vi "SetSMOState.vi"(8 "error in (no error)":errorcluster, 10 "SMO State":T1, 11 "SMO in":refnum<class "SMO.lvclass">) -> (0 "error out":errorcluster, 3 "SMO out":refnum<class "SMO.lvclass">)   [LabVIEW 2021, in "smo.lvlib" / "SMO.lvclass"]
uses:
  SMO.lvclass
  Typedefs/SMOState --Enum.ctl
  SMO.lvclass/SMO.ctl
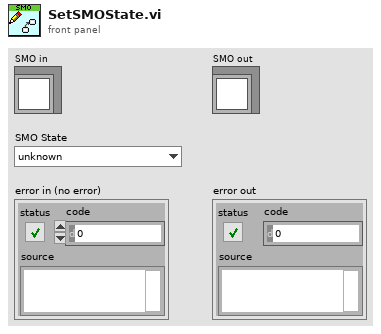
[diagram p1: front panel]
types:
  T1 = typedef "smo.lvlib/SMO.lvclass/SMOState --Enum.ctl" = enum16{"unknown", "Created", "Started", "Stopped"}
  T2 = typedef "smo.lvlib/SMO.lvclass/PrivateData--Ref.ctl" = refnum<data-value>
  T3 = typedef "smo.lvlib/SMO.lvclass/PrivateData--Cluster.ctl" = cluster{"Parent Call":T4, "Registered Processes":T5[], "Sync Notifier":refnum<notifier>, "Process Error Notifier":refnum<notifier>, "Protected Events":T6, "Public Events":T7, "SMO State":T1, "[Attributes]":variant, "Launcher Close":refnum<notifier>, "Caller Watchdog":refnum<queue>, "Accessibility":T8, "NbStaticDependencies":u32}
  T4 = typedef "smo.lvlib/SMO.lvclass/Parent Call--Enum.ctl" = enum16{"Allows parent to run", "Does not request parent to run"}
  T5 = typedef "smo.lvlib/SMO.lvclass/RegisteredProcessData--Cluster.ctl" = cluster{"Name":string, "Static VI Ref":refnum<vi>, "Running":bool, "NotifierRef":u32}
  T6 = typedef "smo.lvlib/SMO.lvclass/Protected Events.ctl" = cluster{"StopProcesses":refnum<user-event>, "AbortProcesses":refnum<user-event>, "Config Changed":refnum<user-event>, "Dependency":refnum<user-event>}
  T7 = typedef "smo.lvlib/SMO.lvclass/Public Events.ctl" = cluster{"Error":refnum<user-event>, "State":refnum<user-event>, "Reserve State":refnum<user-event>}
  T8 = typedef "smo.lvlib/SMO.lvclass/Accessibility--Cluster.ctl" = cluster{"Lock Key":string, "Reserve State":T9}
  T9 = typedef "smo.lvlib/SMO.lvclass/Reserve State--Enum.ctl" = enum16{"Unreserved", "Reserved", "Self-locked"}
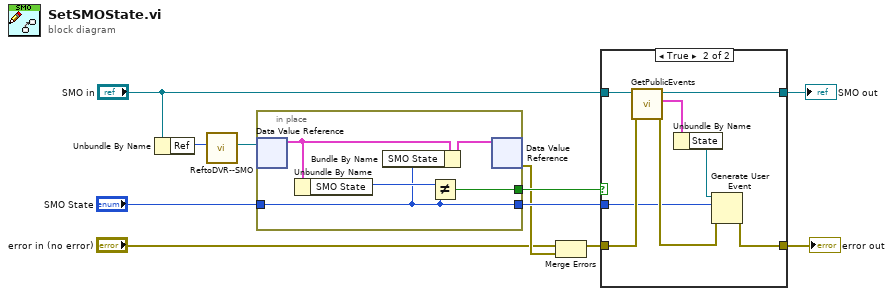
[diagram p0: block diagram]
diagram:
  n1 = Unbundle By Name("SMO in") -> ("Ref"=w6:u32)
  n2 = call "ReftoDVR--SMO.vi"("Ref"=w6) -> ("Ref"=w5:T2)  [unwired: 10 in]
  n3 = in-place {
    in-place-border: "SMO State" -> [w13]
    in-place-border: [w13] -> w8
    in-place-border: [w12] -> w7
    n4 = in-place-dvr #1(w5) -> (w16:T3)  [unwired: 1 out]
    n5 = Unbundle By Name(w16) -> ("SMO State"=w14:T1)
    n6 = Bundle By Name(cluster=w16, "SMO State"=w13) -> (w15:T3)
    n7 = Not Equal?(x=w14, y=w13) -> (x != y?=w12:bool)
    n8 = in-place-dvr #1(w15) -> (w3:errorcluster)  [unwired: 1 out]
  }
  n9 = Merge Errors("error in (no error)", w3) -> (w1:errorcluster)
  n10 = case shown="True" w7 {
    tunnel: [w17 w19] -> w11
    tunnel: [w18 w25] -> w10
    tunnel: "SMO in" -> [w18 w23]
    tunnel: w1 -> [w17 w22]
    tunnel: w8 -> [_ w21]
    frame False {
    }
    frame True {
      n11 = call "GetPublicEvents.vi"("error in (no error)"=w22, "SMO"=w23) -> ("error out"=w24:errorcluster, "Public Events"=w26:T7, "SMO out"=w25:refnum<class "SMO.lvclass">)  [unwired: 7 in]
      n12 = Unbundle By Name(w26) -> ("State"=w20:refnum<user-event>)
      n13 = Generate User Event(user event=w20, event data cluster=w21, error in=w24) -> (error out=w19:errorcluster)  [unwired: 1 in, 1 out]
    }
  }
  "error out" <- w11
  "SMO out" <- w10
